vi "Test Tuner Type.vi"() -> ()   [LabVIEW 2015]
doc: "Created IvanLis by LabVIEW Portal\nProfile: http://labviewportal.org/memberlist.php?mode=viewprofile&u=987\neMail: IvanLisanov@gMail.com\nTelegram: https://t.me/IvanLis"
uses:
  RTL-SDR Class/TypeDef/Tuner Type.ctl
  RTL-SDR Class/RTL-SDR.lvclass
panel:
  out "function return":i32
  out "Tuner Type":T1
  in  "tuner type":bool
  in  "Device Index":u32=1
  in  "Open":bool
  in  "stop":bool
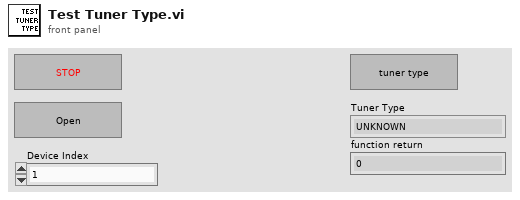
[diagram p1: front panel]
types:
  T1 = typedef "RTL-SDR.lvclass/Tuner Type.ctl" = enum16{"UNKNOWN", "E4000", "FC0012", "FC0013", "FC2580", "R820T", "R828D"}
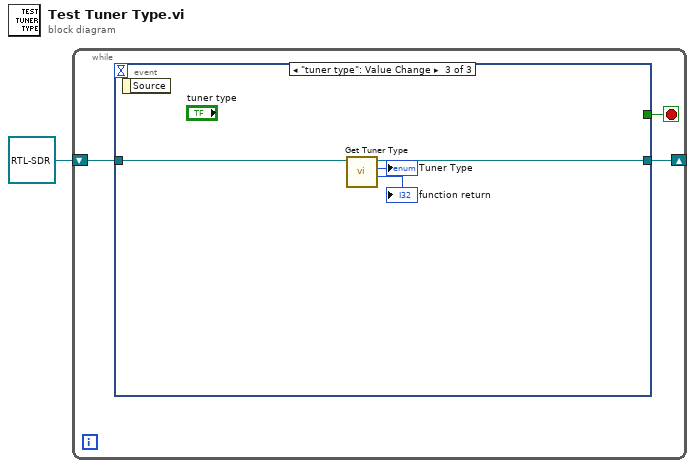
[diagram p0: block diagram]
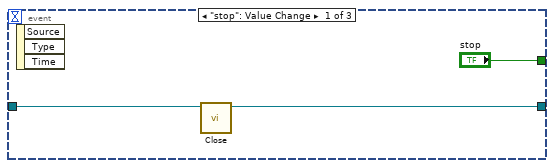
[diagram p2: hidden frame]
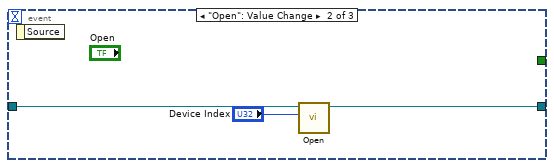
[diagram p3: hidden frame]
diagram:
  n1 = while {
    shift-right: [w2] -> _
    shift-left: refnum<class "RTL-SDR.lvclass"> refnum ("RTL-SDR in") -> [w3]
    stop <- w4 stop-if-true
    n2 = event shown="[2] \"tuner type\": Value Change" {
      selector: _ -> [_ _ _]
      dyn-events: _ -> [_ _ _]
      timeout: _ -> [_ _ _]
      tunnel: ["stop" _ _] -> w4
      tunnel: w3 -> [w6 w10 w14]
      tunnel: [w5 w9 w13] -> w2
      event "stop": Value Change {
        n3 = event-data() -> ()  [unwired: 1 in, 3 out]
        n4 = call "Close.vi"("RTL-SDR in"=w6) -> ("RTL-SDR out"=w5:refnum<class "RTL-SDR.lvclass">)  [unwired: 8 in, 2 out]
      }
      event "Open": Value Change {
        n5 = event-data() -> ()  [unwired: 1 in, 1 out]
        n6 = call "Open.vi"("Device Index"="Device Index", "RTL-SDR in"=w10) -> ("RTL-SDR out"=w9:refnum<class "RTL-SDR.lvclass">)  [unwired: 7 in, 2 out]
      }
      event "tuner type": Value Change {
        n7 = event-data() -> ()  [unwired: 1 in, 1 out]
        n8 = call "Get Tuner Type.vi"("RTL-SDR in"=w14) -> ("function return"=→"function return":i32, "Tuner Type"=→"Tuner Type":T1, "RTL-SDR out"=w13:refnum<class "RTL-SDR.lvclass">)  [unwired: 7 in, 1 out]
      }
    }
  }
